vi "ArduinoHallProbe.vi"() -> ()   [LabVIEW 2014]
uses:
  <vilib>/MakerHub/LINX/Public/Peripherals/Analog/Analog Read 1 Chan.vi
  <vilib>/MakerHub/LINX/Public/Peripherals/Analog/Analog Read N Chans.vi
  <vilib>/MakerHub/LINX/Private/Local IO/LinxAnalogRead.vi
  <vilib>/MakerHub/LINX/Public/Utilities/Check Channel.vi
  <vilib>/MakerHub/LINX/Public/Utilities/Open Serial.vi
  <vilib>/MakerHub/LINX/Private/Utilties/Generate Error.vi
  <vilib>/MakerHub/LINX/LMH-LINX.lvlib
panel:
  in  "Sample Frequency (Hz)":u32
  in  "Analog Pin to Read":i32 min=0 max=5 step=1
  in  "VISA resource name":refnum<visa-resource-name>="COM5"
  in  "stop":bool
  out "Magnetic Field":dbl(graph)
  out "Voltage":dbl
  out "Device Name":string
  out "Error In":errorcluster
  out "Error Out":errorcluster={"status"=FALSE, "code"=1073676294, "source"="VISA Read in LVH-LINX.lvlib:Device.lvlib:Serial Read.vi->LVH-LINX.lvlib:Device.lvlib:Wait For Packet.vi->LVH-LINX.lvlib:Device.lvlib:Send Command.vi->LVH-LINX.lvlib:Device.lvlib:Get DIO Channels.vi->LVH-LINX.lvlib:Device.lvlib:Load Device Config.vi->LVH-LINX.lvlib:Device.lvlib:Initialize Device.vi->LVH-LINX.lvlib:Initialize.vi->Untitled 2"}
  in  "Baud Rate":T1(ring)
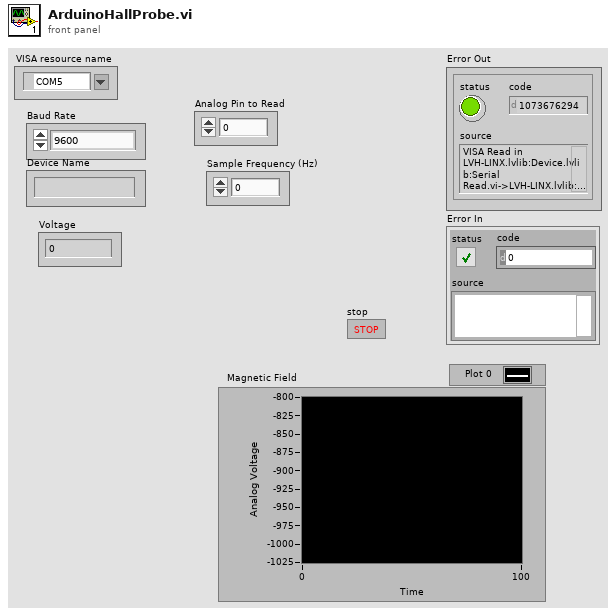
[diagram p1: front panel]
types:
  T1 = enum16{"9600", "14400", "28800", "38400", "57600", "115200"}
  T2 = typedef "LMH-LINX.lvlib/LINX Ref.ctl" = cluster{"IO":T3, "Interface":T4, "LINX Device Config":T5}
  T3 = typedef "LMH-LINX.lvlib/Platform.ctl" = enum16{"Remote", "Local"}
  T4 = typedef "LMH-LINX.lvlib/Interface.ctl" = enum16{"Serial", "TCP"}
  T5 = typedef "LMH-LINX.lvlib/Device.lvlib/LINX Device Config.ctl" = cluster{"Interface":T4, "COM Port":refnum<visa-resource-name>, "TCP Configuration":T6, "Device Family":u8, "Device ID":u8, "Device Name":string, "TCP Ref":refnum<k5>, "Channels":T7}
  T6 = typedef "LMH-LINX.lvlib/Device.lvlib/TCP Config.ctl" = cluster{"IP Address":string, "Port":u16}
  T7 = typedef "LMH-LINX.lvlib/Channels.ctl" = cluster{"DI":u8[], "DO":u8[], "AI":u8[], "AO":u8[], "PWM":u8[], "QE":u8[], "UART":u8[], "I2C 2":u8[], "SPI":u8[], "CAN":u8[], "Servo":u8[], "AI Ref (V)":dbl, "AI Resolution (Bits)":u8, "AO Ref (V)":dbl, "AO Resolution (Bits)":u8}
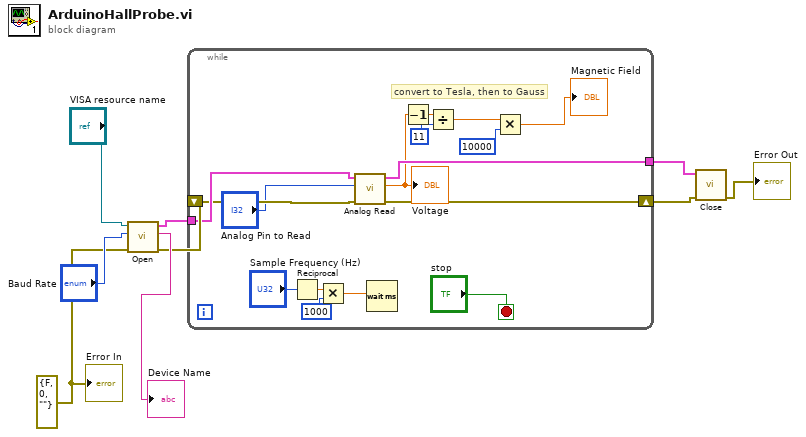
[diagram p0: block diagram]
diagram:
  w1 = errorcluster {"status"=FALSE, "code"=0, "source"=""} ("Error In")
  n1 = call-poly <vilib>:"Open.vi"("Error In"=w1, "Baud Rate Override"="Baud Rate", "Serial Port"="VISA resource name") -> ("Error Out"=w2:errorcluster, "Device Name"=→"Device Name":string, "LINX Resource"=w5:T2)  [unwired: 6 in]
  n2 = while {
    tunnel: [w25] -> w9
    shift-right: [w24] -> w8
    shift-left: w2 -> [w21]
    tunnel: w5 -> [w22]
    stop <- "stop" stop-if-true
    # "convert to Tesla, then to Gauss"
    n3 = Reciprocal(x="Sample Frequency (Hz)") -> (1/x=w18:dbl)
    n4 = Multiply(x=w18, y=1000) -> (x*y=w16:dbl)
    n5 = call-poly <vilib>:"Analog Read.vi"("Error In"=w21, "Analog Channel"="Analog Pin to Read", "LINX Resource"=w22) -> ("Error Out"=w24:errorcluster, "Voltage"=w15:dbl, "LINX Resource"=w25:T2)  [unwired: 5 in, 1 out]
    "Voltage" <- w15
    n6 = Wait (ms)(milliseconds to wait=w16) -> ()  [unwired: 1 out]
    n7 = Decrement(x=w15) -> (x-1=w10:dbl)
    n8 = Divide(x=w10, y=11) -> (x/y=w13:dbl)
    n9 = Multiply(x=w13, y=10000) -> (x*y=→"Magnetic Field":dbl)
  }
  n10 = call <vilib>:"Close.vi"("Error In"=w8, "LINX Resource"=w9) -> ("Error Out"=→"Error Out":errorcluster)  [unwired: 9 in]
  "Error In" <- w1
